vi "créer code EMBALLAGE_ZEBRA_3844Z.vi"(0 "DIVISION":enum16{"FLATPROP", "MEDIC"}(ring)=enum."MEDIC", 1 "N° carton":u8=1, 2 "DATA cmde":T1={"n°article FAS"="12-216C-04521 EQIFIL 417mA 14.4ohm", "n° cmde FAS"="03838/08-01.07.01", "quantité cmde"="100", "ID LIG cmde"="966584", "n° cmde client"="CF-08-0253/2", "nom client"="EMS Electro Medical System", "n° article client"="EL-360", "indice revision client"="03", "société de facturation"="FAS Medic", "langue a utiliser"="FR"}, 3 "Nb total cartons":i32, 9 "Tableau n° valves":string[](array[string])=["112105740008010001", "112105740008010002", "112105740008010003", "112105740008010004", "112105740008010005", "112105740008010006", "112105740008010007", "112105740008010008", "112105740008010009", "112105740008010010", "112105740008010011", "112105740008010012", "112105740008010013", "112105740008010014", "112105740008010015", "112105740008010016", "112105740008010017", "112105740008010018", "112105740008010019", "112105740008010020", "112105740008010021", "112105740008010022", "112105740008010023", "112105740008010024", "112105740008010025", "112105740008010026", "112105740008010027", "112105740008010028", "112105740008010029", "112105740008010030", "112105740008010031", "112105740008010032", "112105740008010033", "112105740008010034", "112105740008010035", "112105740008010036", "112105740008010037", "112105740008010038", "112105740008010039", "112105740008010040", "112105740008010041", "112105740008010042", "112105740008010043", "112105740008010044", "112105740008010045", "112105740008010046", "112105740008010047", "112105740008010048", "112105740008010049", "112105740008010050"], 11 "error in (no error)":errorcluster caption="entrée d'erreur (pas d'erreur)", 12 "Tableau \nlots OUT":string[][](array[string])) -> (6 "chaine  à écrire":string="^XA\n^KL3\n^SC9600,8,N,1,,N\n^PRA\n^LL1428\n^ML888\n^MMC\n^LH100,90\r\r^AFB,1,1^FT0,940^FDDestinataire : EMS Electro Medical System^FS\r^AFB,1,1^FT40,940^FDN§ commande : CF-08-0253/2^FS\r^AFB,1,1^FT80,940^FDQuantit‚ : 50/100^FS\r^AFB,1,1^FT120,940^FDVotre r‚f. : EL-360^FS\r^AFB,1,1^FT200,940^FDN§ valves :^FS\r^AFB,1,1^FT235,905^FD(P/N)^FS\r\r^FT588,30\n^BY2,2.0\n^BCI,80,N,N,N\n^FDEL-360 03 08010801 50^FS\r^A0I,30,30^FT441,0^FDEL-360 03 08010801 50^FS\r\r^A0B,24,24^FT200,750^FD  08010001,  08010002,  08010003,  08010004,  08010005^FS\r^A0B,24,24^FT225,750^FD  08010006,  08010007,  08010008,  08010009,  08010010^FS\r^A0B,24,24^FT250,750^FD  08010011,  08010012,  08010013,  08010014,  08010015^FS\r^A0B,24,24^FT275,750^FD  08010016,  08010017,  08010018,  08010019,  08010020^FS\r^A0B,24,24^FT300,750^FD  08010021,  08010022,  08010023,  08010024,  08010025^FS\r^A0B,24,24^FT325,750^FD  08010026,  08010027,  08010028,  08010029,  08010030^FS\r^A0B,24,24^FT350,750^FD  08010031,  08010032,  08010033,  08010034,  08010035^FS\r^A0B,24,24^FT375,750^FD  08010036,  08010037,  08010038,  08010039,  08010040^FS\r^A0B,24,24^FT400,750^FD  08010041,  08010042,  08010043,  08010044,  08010045^FS\r^A0B,24,24^FT425,750^FD  08010046,  08010047,  08010048,  08010049,  08010050^FS\r\r^FT465,940\n^GB0,800,3^FS\n\n^FT650,940\n^BXB,6,0\n^FD12-216C-04521 EQIFIL 417mA 14.4ohm;03838/08-01.07.01;1/2^FS\r^AFB,1,1^FT525,760^FDN§ article FAS :^FS\r^A0B,30,30^FT560,760^FD12-216C-04521 EQIFIL 417mA 14.4ohm^FS\r^AFB,1,1^FT595,760^FDN§ commande FAS :^FS\r^A0B,30,30^FT630,760^FD03838/08-01.07.01^FS\r^AFB,1,1^FT665,760^FDCarton : ^FS\r^A0B,30,30^FT665,616^FD1/2^FS\r\r^PQ1\n^XZ\r", 8 "Dec.Droite":string="^LH70,20", 10 "n°article FAS":string, 15 "error out":errorcluster caption="sortie d'erreur")   [LabVIEW 2020]
doc: "Crée le code à envoyer à l'imprimante\nFormat : Carton 1/1 dans le code bar 2D"
uses:
  Modules/FS/60_FS_Controles/60_FS_SetGet.ctl
panel:
  out "S122.0009":bool
  out "RETOUR ?":bool
  out "ligne10":string=" 08010046,  08010047,  08010048,  08010049,  08010050"
  out "ligne9":string=" 08010041,  08010042,  08010043,  08010044,  08010045"
  out "ligne8":string=" 08010036,  08010037,  08010038,  08010039,  08010040"
  out "ligne7":string=" 08010031,  08010032,  08010033,  08010034,  08010035"
  out "ligne6":string=" 08010026,  08010027,  08010028,  08010029,  08010030"
  out "ligne5":string=" 08010021,  08010022,  08010023,  08010024,  08010025"
  out "ligne4":string=" 08010016,  08010017,  08010018,  08010019,  08010020"
  out "ligne3":string=" 08010011,  08010012,  08010013,  08010014,  08010015"
  out "ligne2":string=" 08010006,  08010007,  08010008,  08010009,  08010010"
  out "ligne1":string=" 08010001,  08010002,  08010003,  08010004,  08010005"
  out "Ref client":string="EL-360"
  out "Quantité":string="50/100"
  out "carton":string="1/2"
  out "N° cmde client":string="CF-08-0253/2"
  out "Nom client":string="EMS Electro Medical System"
  out "nom valve FAS":string="12-216C-04521 EQIFIL 417mA 14.4ohm"
  out "n° commande FAS":string="03838/08-01.07.01"
  out "nom sous code bar client":string="EL-360 03 08010801 50"
  # "^XA\n^KL3\n^SC9600,8,N,1,,N\n^PRA\n^LL976\n^ML592\n^LH25,25\n\n^ADB,1,1^FT25,704^FDDestinataire :  EMS Electro Medical System^FS\n^ADB,1,1^FT50,704^FDN§ commande : CF-08-0253/2^FS\n^ADB,1,1^FT75,704^FDCarton : 1/2^FS\n^ADB,1,1^FT100,704^FDQuantit‚ : 50/100^FS\n^ADB,1,1^FT125,704^FDVotre r‚f. : EL-360^FS\n\n^ADB,1,1^FT180,704^FDN§ valves :^FS\n^ADB,1,1^FT205,678^FD(P/N)^FS\n^A0B,18,18^FT180,568^FD 08120001,  08120002,  08120003,  08120004,  08120005^FS\n^A0B,18,18^FT198,568^FD 08120006,  08120007,  08120008,  08120009,  08120010^FS\n^A0B,18,18^FT216,568^FD 08120011,  08120012,  08120013,  08120014,  08120015^FS\n^A0B,18,18^FT234,568^FD 08120016,  08120017,  08120018,  08120019,  08120020^FS\n^A0B,18,18^FT252,568^FD 08120021,  08120022,  08120023,  08120024,  08120025^FS\n^A0B,18,18^FT270,568^FD 08120026,  08120027,  08120028,  08120029,  08120030^FS\n^A0B,18,18^FT288,568^FD 08120031,  08120032,  08120033,  08120034,  08120035^FS\n^A0B,18,18^FT306,568^FD 08120036,  08120037,  08120038,  08120039,  08120040^FS\n^A0B,18,18^FT324,568^FD 08120041,  08120042,  08120043,  08120044,  08120045^FS\n^A0B,18,18^FT342,568^FD 08120046,  08120047,  08120048,  08120049,  08120050^FS\n\n^FT370,708\n^GB0,565,3^FS\n\n^FT501,708\n^BXB,4,0\n^FD12-216C-04521 EQIFIL 417mA 14.4ohm     03838/08-07.01.01^FS\n\n^ADB,1,1^FT413,568^FDN§ article FAS :^FS\n^AQB,1,1^FT443,568^FD12-216C-04521 EQIFIL 417mA 14.4ohm^FS\n^ADB,1,1^FT470,568^FDN§ commande FAS :^FS\n^AQB,1,1^FT500,568^FD03838/08-07.01.01^FS\n\n^FT352,40\n^BY1,2.0\n^BCI,56,N,N,N\n^FDEL-360 03 08120812 50^FS\n^AQI,1,1^FT352,10^FDEL-360 03 08120812 50^FS\n\n^PQ1\n^XZ"
  # "Destinataire:"
  # "N°commande :"
  # "Quantité:"
  # "Votre ref.:"
  # "N° valves :\n(P/N)"
  # "N°article FAS:"
  # "N°commande FAS:"
  # "Carton :"
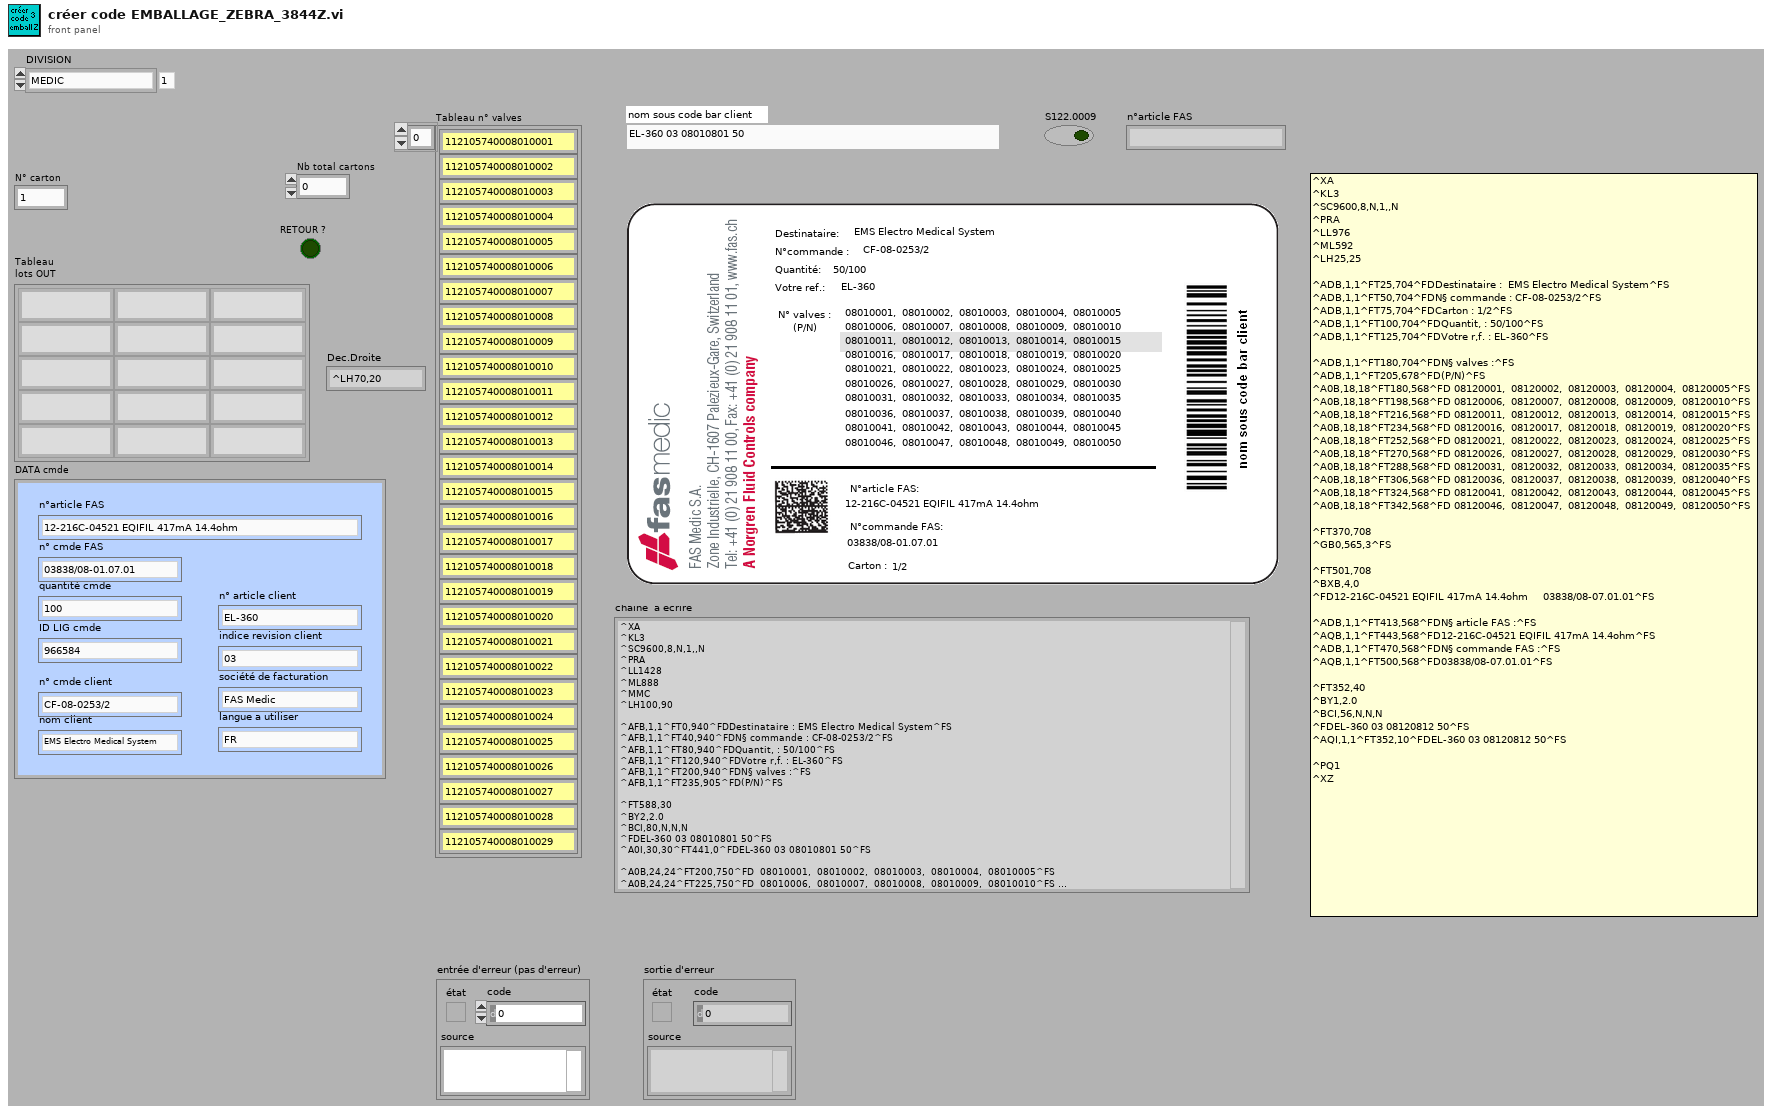
[diagram p1: front panel]
types:
  T1 = typedef "DATA commande.ctl" = cluster{"n°article FAS":string, "n° cmde FAS":string, "quantité cmde":string, "ID LIG cmde":string, "n° cmde client":string, "nom client":string, "n° article client":string, "indice revision client":string, "société de facturation":string, "langue a utiliser":string}
  T2 = typedef "60_FS_SetGet.ctl" = enum16{"set", "get"}
  T3 = typedef "Emballage_BDD_param_Produit.ctl" = cluster{"No_Valve_FAS":string, "suffixe":string, "designation":string, "indice_produit":string, "code_barre_fixe":string, "affiche_code_barre_client":string, "affiche_no_client":string, "Nb_vlve_par_carton":u16, "melange_des_lots_possible":string, "id_article":string, "Indice_Rev":string, "Famille":string, "date":string, "code_barre_fixe_Fin":string, "Longeur_No_Serie":string}
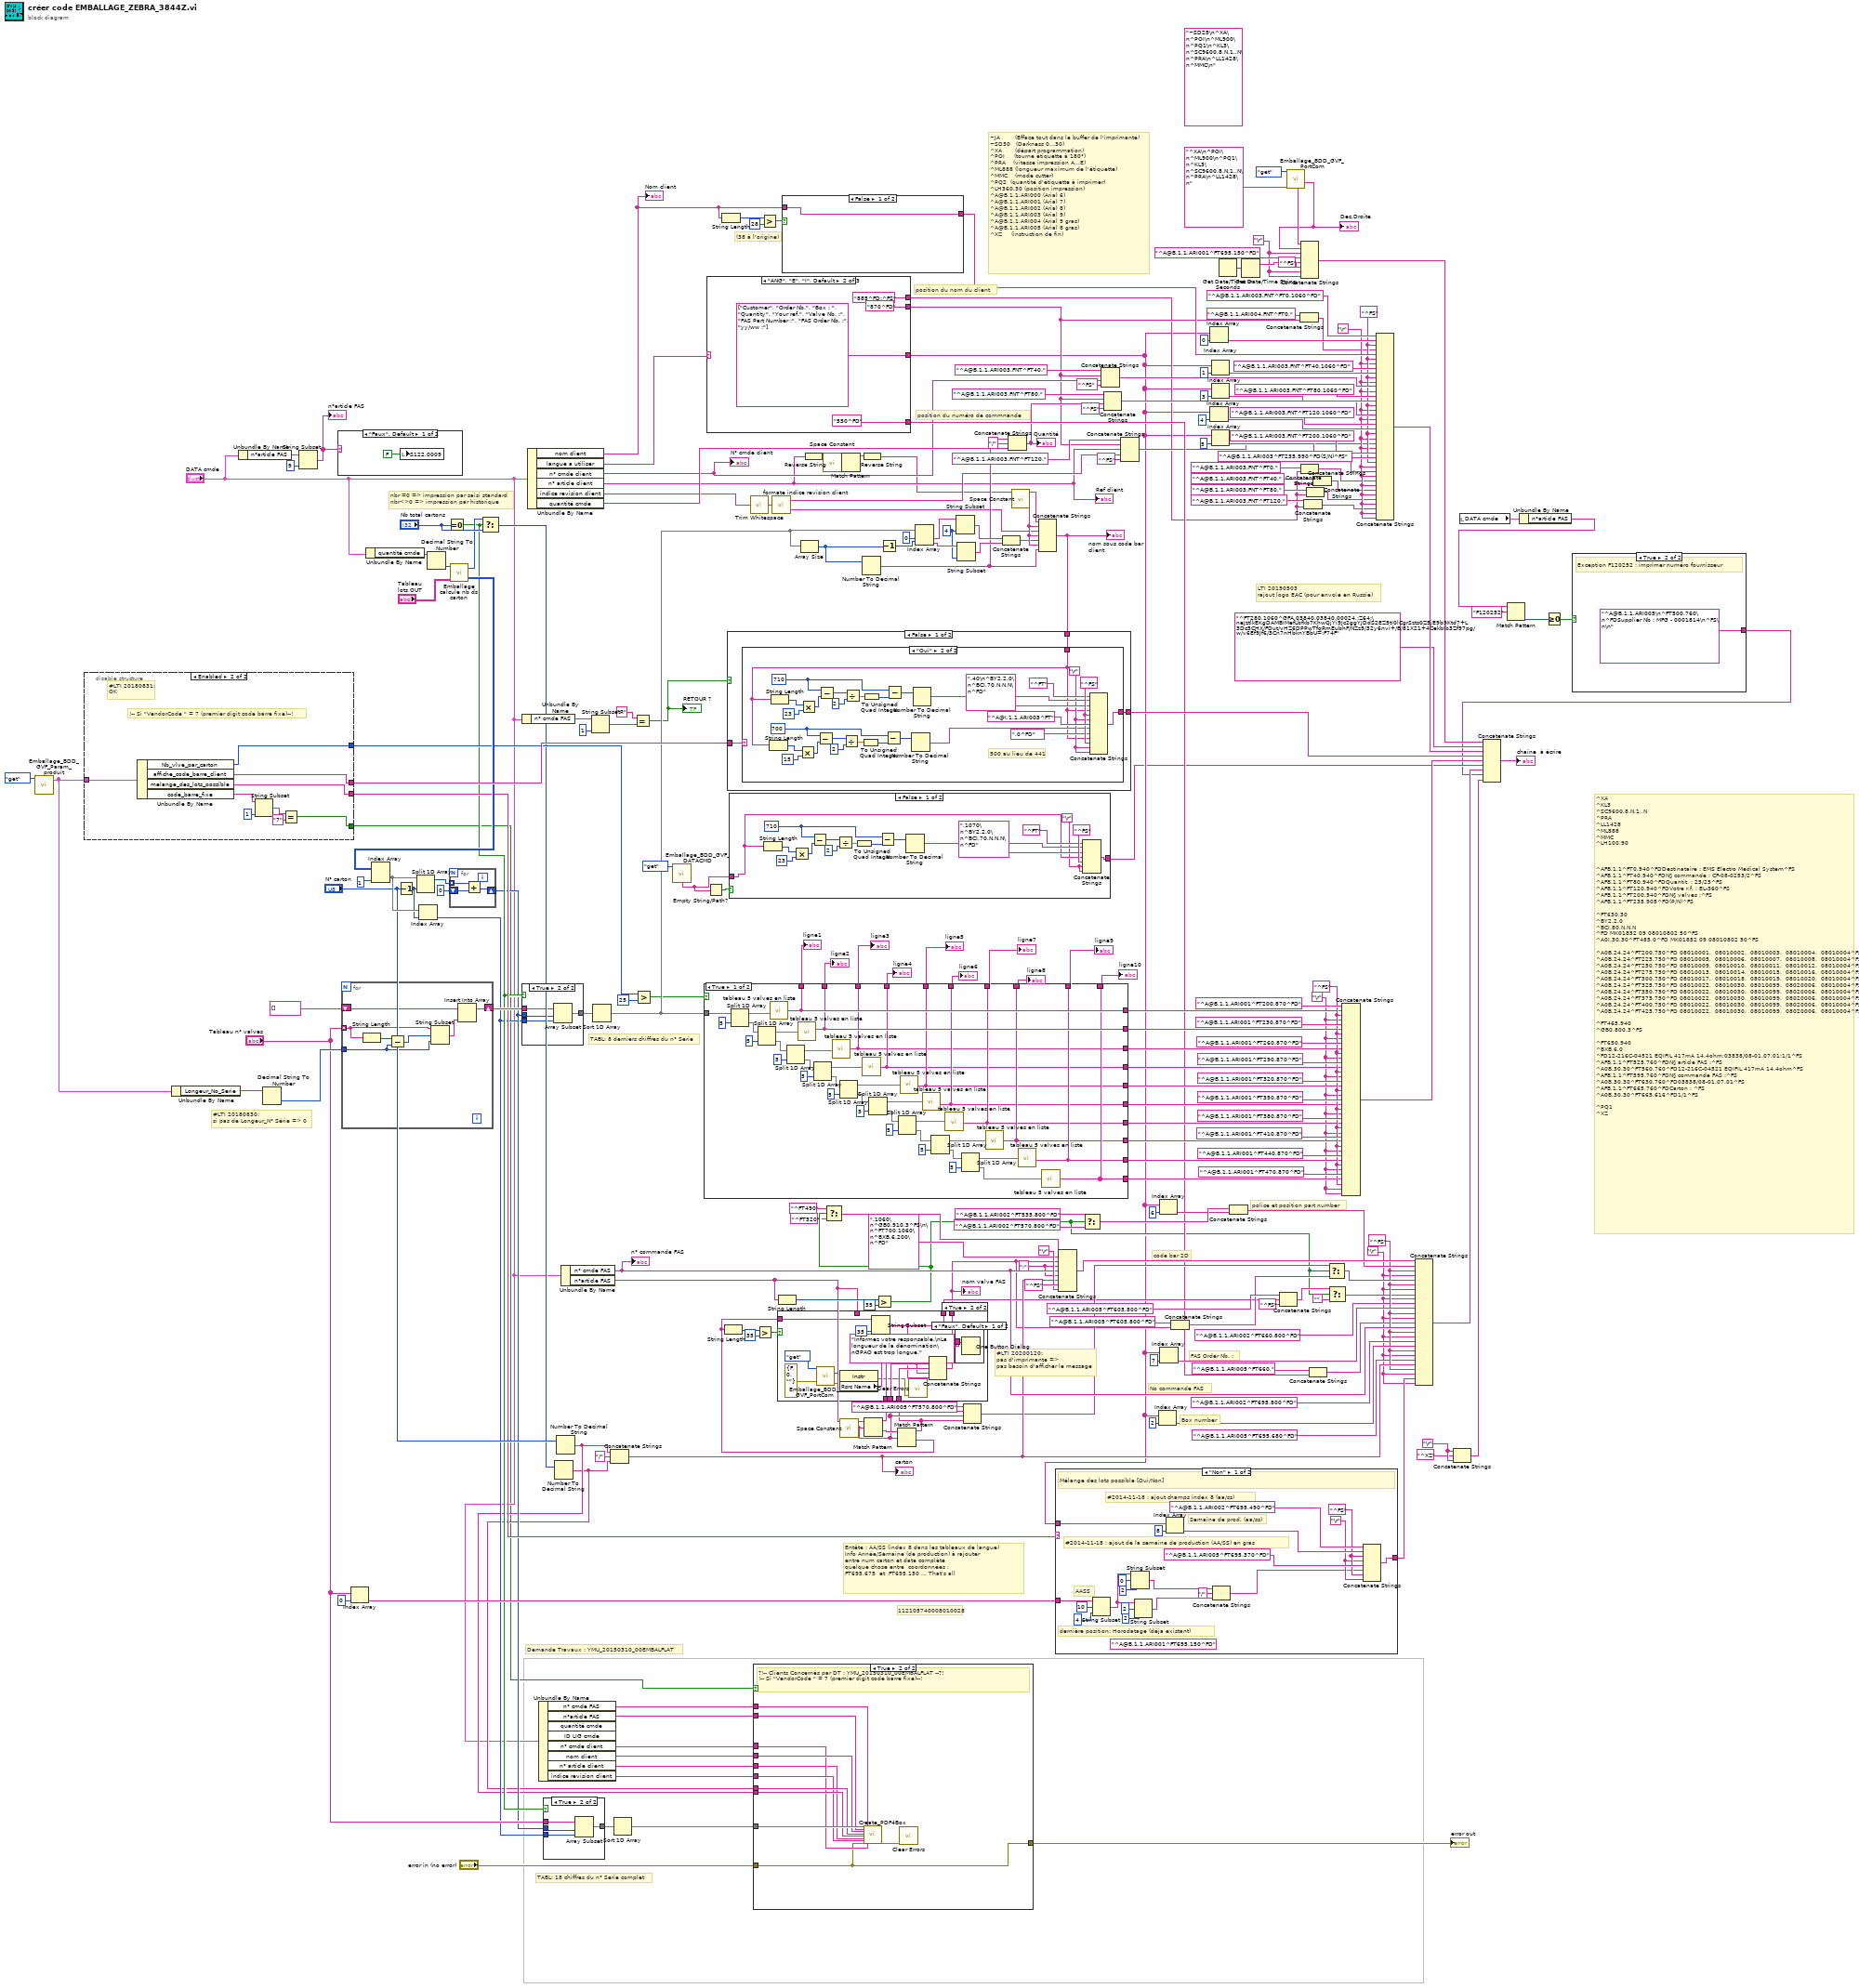
[diagram p0: block diagram]
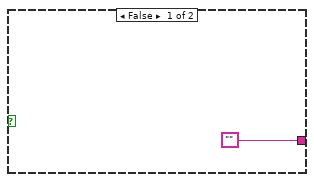
[diagram p2: hidden frame]
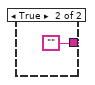
[diagram p3: hidden frame]
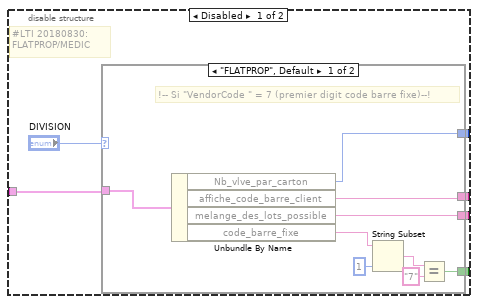
[diagram p4: hidden frame]
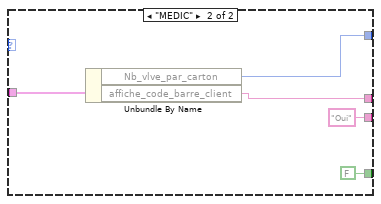
[diagram p5: hidden frame]
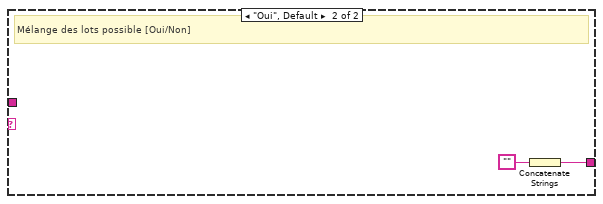
[diagram p8: hidden frame]
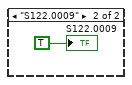
[diagram p9: hidden frame]
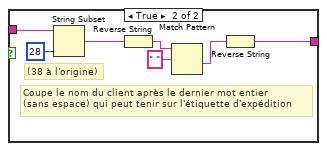
[diagram p11: hidden frame]
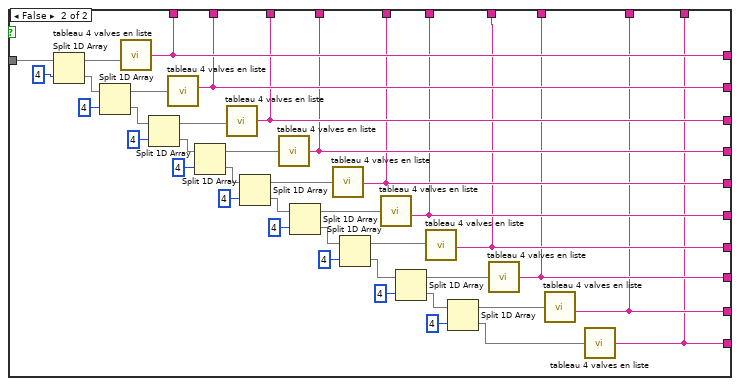
[diagram p14: hidden frame]
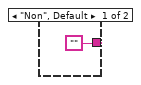
[diagram p15: hidden frame]
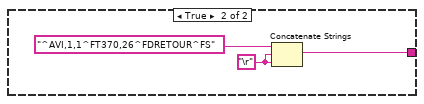
[diagram p16: hidden frame]
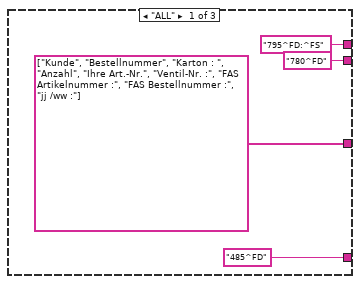
[diagram p17: hidden frame]
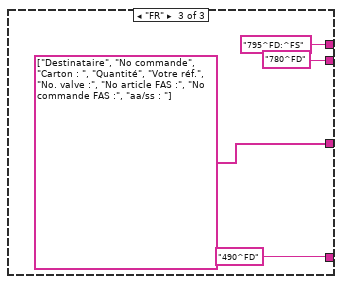
[diagram p18: hidden frame]
diagram:
  (unwired) "~SD25\n^XA\n^POI\n^ML900\n^PQ1\n^KL3\n^SC9600,8,N,1,,N\n^PRA\n^LL1428\n^MMC\n"
  w119 = "\r"
  w41 = "\r"
  w123 = "^FS"
  w144 = ";"
  w203 = "^FS"
  w164 = "\r"
  w94 = "^FS"
  w93 = "\r"
  w48 = "\r"
  w234 = 4 ("longueur (reste)")
  # "#LTI 20200120:\npas d'imprimante =>\npas besoin d'afficher le message"
  # "LTI 20190503\nrajout logo EAC (pour envoie en Russie)"
  # "#LTI 20180830:\nsi pas de Longeur_N° Série => 0"
  # "Demande Travaux : YMU_20150310_00EMBALFLAT"
  # "TABL: 18 chiffres du n° Serie complet"
  # "TABL: 8 derniers chiffres du n° Serie"
  # "112105740008010028"
  # "Entête : AA/SS (index 8 dans les tableaux de langue)\nInfo Année/Semaine (de production) à rajouter \nentre num carton et date complète\nquelque chose entre  coordonnées :      \nFT695,675  et  FT695,150 ... That's all"
  # "(38 à l'origine)"
  # "nbr =0 => impression par saisi standard\nnbr<>0 => impression par historique"
  # "position du numéro de commnande"
  # "position du nom du client"
  # "Box number"
  # "No commande FAS"
  # "FAS Order Nb. :"
  # "police et position part number"
  # "code bar 2D"
  # "~JA        (Efface tout dans le buffer de l'imprimante)\n~SD30   (Darkness 0...30)\n^XA       (départ programmation)\n^POI     (tourne étiquette à 180°)\n^PRA    (vitesse impression A...E)\n^ML888 (longueur maximum de l'étiquette)\n^MMC    (mode cutter)\n^PQ2  (quantité d'étiquette à imprimer)\n^LH360,30 (position impression)\n^A@B,1,1,ARI000 (Arial 6)\n^A@B,1,1,ARI001 (Arial 7)\n^A@B,1,1,ARI002 (Arial 8)\n^A@B,1,1,ARI003 (Arial 9)\n^A@B,1,1,ARI004 (Arial 9 gras)\n^A@B,1,1,ARI005 (Arial 8 gras)\n^XZ     (instruction de fin)"
  # "^XA\n^KL3\n^SC9600,8,N,1,,N\n^PRA\n^LL1428\n^ML888\n^MMC\n^LH100,90\n\n\n\n^AFB,1,1^FT0,940^FDDestinataire : EMS Electro Medical System^FS\n^AFB,1,1^FT40,940^FDN§ commande : CF-08-0253/2^FS\n^AFB,1,1^FT80,940^FDQuantit‚ : 25/25^FS\n^AFB,1,1^FT120,940^FDVotre r‚f. : EL-360^FS\n^AFB,1,1^FT200,940^FDN§ valves :^FS\n^AFB,1,1^FT235,905^FD(P/N)^FS\n\n^FT630,30\n^BY2,2.0\n^BCI,80,N,N,N\n^FD MK01852 09 08010802 50^FS\n^A0I,30,30^FT485,0^FD MK01852 09 08010802 50^FS\n\n^A0B,24,24^FT200,750^FD 08010001,  08010002,  08010003,  08010004,  08010004^FS\n^A0B,24,24^FT225,750^FD 08010005,  08010006,  08010007,  08010008,  08010004^FS\n^A0B,24,24^FT250,750^FD 08010009,  08010010,  08010011,  08010012,  08010004^FS\n^A0B,24,24^FT275,750^FD 08010013,  08010014,  08010015,  08010016,  08010004^FS\n^A0B,24,24^FT300,750^FD 08010017,  08010018,  08010019,  08010020,  08010004^FS\n^A0B,24,24^FT325,750^FD 08010022,  08010030,  08010099,  08020006,  08010004^FS\n^A0B,24,24^FT350,750^FD 08010022,  08010030,  08010099,  08020006,  08010004^FS\n^A0B,24,24^FT375,750^FD 08010022,  08010030,  08010099,  08020006,  08010004^FS\n^A0B,24,24^FT400,750^FD 08010022,  08010030,  08010099,  08020006,  08010004^FS\n^A0B,24,24^FT425,750^FD 08010022,  08010030,  08010099,  08020006,  08010004^FS\n\n^FT465,940\n^GB0,800,3^FS\n\n^FT650,940\n^BXB,6,0\n^FD12-216C-04521 EQIFIL 417mA 14.4ohm;03838/08-01.07.01;1/1^FS\n^AFB,1,1^FT525,760^FDN§ article FAS :^FS\n^A0B,30,30^FT560,760^FD12-216C-04521 EQIFIL 417mA 14.4ohm^FS\n^AFB,1,1^FT595,760^FDN§ commande FAS :^FS\n^A0B,30,30^FT630,760^FD03838/08-01.07.01^FS\n^AFB,1,1^FT665,760^FDCarton : ^FS\n^A0B,30,30^FT665,616^FD1/1^FS\n\n^PQ1\n^XZ"
  n1 = call "Emballage_BDD_GVF_Param_produit.vi"("Énum"=enum16{"set", "get"}."get") -> ("CLS_param_produit"=w17:T3)  [unwired: 7 in, 3 out]
  n2 = disable-structure shown="Enabled" {
    disable-tunnel: [w245 w261] -> w189
    disable-tunnel: [w244 w260] -> w150
    disable-tunnel: [w243 w262] -> w44
    disable-tunnel: [w242 w264] -> w21
    disable-tunnel: w17 -> [w241 w263]
    frame Disabled {
      # "#LTI 20180830:\nFLATPROP/MEDIC"
      n3 = case shown="\"FLATPROP\", Default" "DIVISION" {
        tunnel: [w253 w256] -> w245
        tunnel: [w254 w255] -> w244
        tunnel: w241 -> [w252 w257]
        tunnel: [w251 "Oui" ("Mélange des lots posiible [Oui/Non]")] -> w243
        tunnel: [w246 FALSE] -> w242
        frame "FLATPROP", Default {
          # "!-- Si \"VendorCode \" = 7 (premier digit code barre fixe)--!"
          n4 = Unbundle By Name(w252) -> ("Nb_vlve_par_carton"=w254:u16, "affiche_code_barre_client"=w253:string, "melange_des_lots_possible"=w251:string, "code_barre_fixe"=w250:string)
          n5 = String Subset(string=w250, length (rest)=1 ("longueur (reste)")) -> (substring=w248:string)  [unwired: 1 in]
          n6 = Equal?(x=w248, y="7") -> (x = y?=w246:bool)
        }
        frame "MEDIC" {
          n7 = Unbundle By Name(w257) -> ("Nb_vlve_par_carton"=w255:u16, "affiche_code_barre_client"=w256:string)
        }
      }
    }
    frame Enabled {
      # "#LTI 20180831:\nOK"
      # "!-- Si \"VendorCode \" = 7 (premier digit code barre fixe)--!"
      n8 = Unbundle By Name(w263) -> ("Nb_vlve_par_carton"=w260:u16, "affiche_code_barre_client"=w261:string, "melange_des_lots_possible"=w262:string, "code_barre_fixe"=w268:string)
      n9 = String Subset(string=w268, length (rest)=1 ("longueur (reste)")) -> (substring=w266:string)  [unwired: 1 in]
      n10 = Equal?(x=w266, y="7") -> (x = y?=w264:bool)
    }
  }
  n11 = Unbundle By Name(w17) -> ("Longeur_No_Serie"=w16:string)
  n12 = Unbundle By Name("DATA cmde") -> ("n°article FAS"=w47:string)
  n13 = Decimal String To Number(string=w16) -> (number=w50:i32)  [unwired: 2 in, 1 out]
  n14 = String Subset(string=w47, length (rest)=9 ("longueur (reste)")) -> (substring=w45:string)  [unwired: 1 in]
  "n°article FAS" <- w45
  n15 = case shown="\"Faux\", Default" w45 {
    frame "Faux", Default {
      n16 = local write "S122.0009"(FALSE ("S122.0009")) -> ()
    }
    frame "S122.0009" {
      "S122.0009" <- TRUE ("S122.0009")
    }
  }
  n17 = for {
    tunnel: "Tableau n° valves" -> [w274] mode=indexing
    shift-right: [w276] -> w185
    shift-left: string[] [] -> [w275]
    tunnel: w50 -> [w271]
    n18 = String Length(string=w274) -> (length=w273:i32)
    n19 = Subtract(x=w273, y=w271) -> (x-y=w272:i32)
    n20 = String Subset(string=w274, offset (0)=w272, length (rest)=w271) -> (substring=w277:string)
    n21 = Insert Into Array(array=w275, new element=w277) -> (w276:string[])  [unwired: 1 in]
  }
  n22 = Index Array(array="Tableau n° valves", index=0 ("indice")) -> (element=w39:string)
  n23 = Unbundle By Name("DATA cmde") -> ("quantité cmde"=w19:string)
  n24 = Decrement(x="N° carton") -> (x-1=w180:u8)
  n25 = Decimal String To Number(string=w19) -> (number=w18:i32)  [unwired: 2 in, 1 out]
  n26 = Equal To 0?(x="Nb total cartons") -> (x = 0?=w36:bool)
  n27 = call "Emballage calcule nb ds carton.vi"("Tableau \nlots OUT"="Tableau \nlots OUT", "Quantité de la cmde"=w18) -> ("Tab n° carton - nb ds carton"=w177:i32[][], "Nb total cartons"=w59:i32)  [unwired: 1 in]
  n28 = Index Array(array=w177, index (col)=1 ("indice désactivé (col)")) -> (element=w181:i32[])  [unwired: 1 in]
  n29 = Split 1D Array(array=w181, index=w180) -> (first subarray=w182:i32[])  [unwired: 1 out]
  n30 = Index Array(array=w181, index=w180) -> (element=w34:i32)
  n31 = for {
    tunnel: w182 -> [w280] mode=indexing
    shift-right: [w278] -> w35
    shift-left: 0 -> [w279]
    n32 = Add(x=w280, y=w279) -> (x+y=w278:i32)
  }
  n33 = Select(t=w59, s=w36, f="Nb total cartons") -> (s? t:f=w58:i32)
  n34 = Unbundle By Name("DATA cmde") -> ("n° cmde FAS"=w149:string)
  n35 = case shown="True" w36 {
    tunnel: w185 -> [w281 w285]
    tunnel: [w281 w284] -> w184
    tunnel: w35 -> [_ w283]
    tunnel: w34 -> [_ w282]
    frame False {
    }
    frame True {
      n36 = Array Subset(array=w285, index=w283, length=w282) -> (w284:string[])
    }
  }
  n37 = Unbundle By Name("DATA cmde") -> ("nom client"=w112:string, "langue a utiliser"=w191:string, "n° cmde client"=w100:string, "n° article client"=w55:string, "indice revision client"=w56:string, "quantité cmde"=w190:string)
  "Nom client" <- w112
  "N° cmde client" <- w100
  "Ref client" <- w55
  n38 = Unbundle By Name("DATA cmde") -> ("n° cmde FAS"=w29:string, "n°article FAS"=w28:string, "n° cmde client"=w26:string, "nom client"=w22:string, "n° article client"=w25:string, "indice revision client"=w27:string)  [unwired: 2 out]
  n39 = case shown="True" w36 {
    tunnel: "Tableau n° valves" -> [w286 w290]
    tunnel: [w286 w289] -> w38
    tunnel: w35 -> [_ w288]
    tunnel: w34 -> [_ w287]
    frame False {
    }
    frame True {
      n40 = Array Subset(array=w290, index=w288, length=w287) -> (w289:string[])
    }
  }
  n41 = Number To Decimal String(number=w58) -> (decimal integer string=w31:string)  [unwired: 1 in]
  n42 = Number To Decimal String(number="N° carton") -> (decimal integer string=w32:string)  [unwired: 1 in]
  n43 = Unbundle By Name("DATA cmde") -> ("n° cmde FAS"=w175:string, "n°article FAS"=w107:string)
  "n° commande FAS" <- w175
  n44 = String Subset(string=w149, length (rest)=1 ("longueur (reste)")) -> (substring=w146:string)  [unwired: 1 in]
  n45 = Sort 1D Array(array=w184) -> (sorted array=w178:string[])
  n46 = Concatenate Strings(w32, "/", w31) -> (w141:string)
  "carton" <- w141
  n47 = Sort 1D Array(array=w38) -> (sorted array=w33:string[])
  n48 = Equal?(x="R", y=w146) -> (x = y?=w147:bool)
  "RETOUR ?" <- w147
  n49 = Greater?(x=w150, y=u16 25) -> (0:w152:bool)
  n50 = call "Emballage_BDD_GVF_DATACMD.vi"("SetGet"=60_FS_SetGet."get") -> ("NO_ARTICLE_JDE"=w10:string)  [unwired: 7 in, 7 out]
  n51 = case shown="True" w152 {
    tunnel: w178 -> [w301 w339]
    tunnel: [w300 w338] -> w174
    tunnel: [w299 w337] -> w173
    tunnel: [w291 w336] -> w172
    tunnel: [w298 w329] -> w171
    tunnel: [w297 w330] -> w170
    tunnel: [w296 w331] -> w169
    tunnel: [w295 w332] -> w168
    tunnel: [w294 w333] -> w167
    tunnel: [w293 w334] -> w166
    tunnel: [w292 w335] -> w165
    tunnel: [w300 w338] -> w162
    tunnel: [w299 w337] -> w161
    tunnel: [w298 w329] -> w160
    tunnel: [w297 w330] -> w159
    tunnel: [w296 w331] -> w158
    tunnel: [w295 w332] -> w157
    tunnel: [w294 w333] -> w156
    tunnel: [w293 w334] -> w155
    tunnel: [w292 w335] -> w154
    tunnel: [w291 w336] -> w153
    frame True {
      n52 = Split 1D Array(array=w301, index=5 ("indice")) -> (first subarray=w319:string[], second subarray=w326:string[])
      n53 = Split 1D Array(array=w326, index=5 ("indice")) -> (first subarray=w318:string[], second subarray=w324:string[])
      n54 = call "tableau 5 valves en liste.vi"("Tableau de 5 valves"=w319) -> ("Chaîne de 5 valves"=w300:string)
      n55 = Split 1D Array(array=w324, index=5 ("indice")) -> (first subarray=w317:string[], second subarray=w322:string[])
      n56 = call "tableau 5 valves en liste.vi"("Tableau de 5 valves"=w318) -> ("Chaîne de 5 valves"=w299:string)
      n57 = Split 1D Array(array=w322, index=5 ("indice")) -> (first subarray=w316:string[], second subarray=w320:string[])
      n58 = call "tableau 5 valves en liste.vi"("Tableau de 5 valves"=w317) -> ("Chaîne de 5 valves"=w291:string)
      n59 = Split 1D Array(array=w320, index=5 ("indice")) -> (first subarray=w315:string[], second subarray=w313:string[])
      n60 = call "tableau 5 valves en liste.vi"("Tableau de 5 valves"=w316) -> ("Chaîne de 5 valves"=w292:string)
      n61 = Split 1D Array(array=w313, index=5 ("indice")) -> (first subarray=w312:string[], second subarray=w310:string[])
      n62 = Split 1D Array(array=w310, index=5 ("indice")) -> (first subarray=w309:string[], second subarray=w307:string[])
      n63 = call "tableau 5 valves en liste.vi"("Tableau de 5 valves"=w315) -> ("Chaîne de 5 valves"=w293:string)
      n64 = call "tableau 5 valves en liste.vi"("Tableau de 5 valves"=w312) -> ("Chaîne de 5 valves"=w294:string)
      n65 = Split 1D Array(array=w307, index=5 ("indice")) -> (first subarray=w306:string[], second subarray=w304:string[])
      n66 = call "tableau 5 valves en liste.vi"("Tableau de 5 valves"=w309) -> ("Chaîne de 5 valves"=w295:string)
      n67 = Split 1D Array(array=w304, index=5 ("indice")) -> (first subarray=w303:string[], second subarray=w302:string[])
      n68 = call "tableau 5 valves en liste.vi"("Tableau de 5 valves"=w306) -> ("Chaîne de 5 valves"=w296:string)
      n69 = call "tableau 5 valves en liste.vi"("Tableau de 5 valves"=w303) -> ("Chaîne de 5 valves"=w297:string)
      n70 = call "tableau 5 valves en liste.vi"("Tableau de 5 valves"=w302) -> ("Chaîne de 5 valves"=w298:string)
    }
    frame False {
      n71 = Split 1D Array(array=w339, index=4 ("indice")) -> (first subarray=w357:string[], second subarray=w364:string[])
      n72 = Split 1D Array(array=w364, index=4 ("indice")) -> (first subarray=w356:string[], second subarray=w362:string[])
      n73 = call "tableau 4 valves en liste.vi"("Tableau de 4 valves"=w357) -> ("Chaîne de 5 valves"=w338:string)
      n74 = Split 1D Array(array=w362, index=4 ("indice")) -> (first subarray=w355:string[], second subarray=w360:string[])
      n75 = call "tableau 4 valves en liste.vi"("Tableau de 4 valves"=w356) -> ("Chaîne de 5 valves"=w337:string)
      n76 = Split 1D Array(array=w360, index=4 ("indice")) -> (first subarray=w354:string[], second subarray=w358:string[])
      n77 = call "tableau 4 valves en liste.vi"("Tableau de 4 valves"=w355) -> ("Chaîne de 5 valves"=w336:string)
      n78 = Split 1D Array(array=w358, index=4 ("indice")) -> (first subarray=w353:string[], second subarray=w351:string[])
      n79 = call "tableau 4 valves en liste.vi"("Tableau de 4 valves"=w354) -> ("Chaîne de 5 valves"=w335:string)
      n80 = Split 1D Array(array=w351, index=4 ("indice")) -> (first subarray=w350:string[], second subarray=w348:string[])
      n81 = call "tableau 4 valves en liste.vi"("Tableau de 4 valves"=w353) -> ("Chaîne de 5 valves"=w334:string)
      n82 = Split 1D Array(array=w348, index=4 ("indice")) -> (first subarray=w347:string[], second subarray=w345:string[])
      n83 = call "tableau 4 valves en liste.vi"("Tableau de 4 valves"=w350) -> ("Chaîne de 5 valves"=w333:string)
      n84 = Split 1D Array(array=w345, index=4 ("indice")) -> (first subarray=w344:string[], second subarray=w342:string[])
      n85 = call "tableau 4 valves en liste.vi"("Tableau de 4 valves"=w347) -> ("Chaîne de 5 valves"=w332:string)
      n86 = Split 1D Array(array=w342, index=4 ("indice")) -> (first subarray=w341:string[], second subarray=w340:string[])
      n87 = call "tableau 4 valves en liste.vi"("Tableau de 4 valves"=w344) -> ("Chaîne de 5 valves"=w331:string)
      n88 = call "tableau 4 valves en liste.vi"("Tableau de 4 valves"=w341) -> ("Chaîne de 5 valves"=w330:string)
      n89 = call "tableau 4 valves en liste.vi"("Tableau de 4 valves"=w340) -> ("Chaîne de 5 valves"=w329:string)
    }
  }
  "ligne1" <- w162
  "ligne2" <- w161
  "ligne3" <- w153
  "ligne4" <- w154
  "ligne5" <- w155
  "ligne6" <- w156
  "ligne7" <- w157
  "ligne8" <- w158
  "ligne9" <- w159
  "ligne10" <- w160
  n90 = case shown="\"ANG\", \"E\", \"I\", Default" w191 {
    tunnel: [string[] ["Kunde", "Bestellnummer", "Karton : ", "Anzahl", "Ihre Art.-Nr.", "Ventil-Nr. :", "FAS Artikelnummer :", "FAS Bestellnummer :", "jj /ww :"] string[] ["Customer", "Order Nb.", "Box : ", "Quantity", "Your ref.", "Valve Nb. :", "FAS Part Number :", "FAS Order Nb. :", "yy/ww :"] string[] ["Destinataire", "No commande", "Carton : ", "Quantité", "Votre réf.", "No. valve :", "No article FAS :", "No commande FAS :", "aa/ss : "]] -> w43
    tunnel: ["485^FD" "550^FD" "490^FD"] -> w101
    tunnel: ["795^FD:^FS" "885^FD:^FS" "795^FD:^FS"] -> w78
    tunnel: ["780^FD" "870^FD" "780^FD"] -> w87
    frame "ALL" {
    }
    frame "ANG", "E", "I", Default {
    }
    frame "FR" {
    }
  }
  n91 = Empty String/Path?(string/path=w10) -> (empty?=w11:bool)
  n92 = String Length(string=w112) -> (length=w114:i32)
  n93 = case shown="False" w11 {
    tunnel: [w381 ""] -> w9
    tunnel: w10 -> [w380 _]
    frame False {
      w388 = 710
      w379 = "\r"
      n94 = String Length(string=w380) -> (length=w393:i32)
      n95 = Multiply(x=w393, y=23) -> (x*y=w391:i32)
      n96 = Subtract(x=w388, y=w391) -> (x-y=w390:i32)
      n97 = Divide(x=w390, y=2) -> (x/y=w387:dbl)
      n98 = To Unsigned Quad Integer(1:w387) -> (0:w386:u64)
      n99 = Subtract(x=w388, y=w386) -> (x-y=w385:u64)
      n100 = Number To Decimal String(number=w385) -> (decimal integer string=w382:string)  [unwired: 1 in]
      n101 = Concatenate Strings("^FT", w382, ",1070\n^BY2,2.0\n^BCI,70,N,N,N\n^FD", w380, "^FS", w379, w379) -> (w381:string)
    }
    frame True {
    }
  }
  n102 = call <vilib>:"Trim Whitespace.vi"("string"=w56) -> ("trimmed string"=w57:string)  [unwired: 1 in]
  n103 = case shown="True" w21 {
    tunnel: w33 -> [_ w407]
    tunnel: w32 -> [_ w406]
    tunnel: w31 -> [_ w405]
    tunnel: w29 -> [_ w404]
    tunnel: w28 -> [_ w403]
    tunnel: w22 -> [_ w402]
    tunnel: w27 -> [_ w401]
    tunnel: w26 -> [_ w400]
    tunnel: w25 -> [_ w399]
    tunnel: [w396 w397] -> w24
    tunnel: "error in (no error)" -> [w396 w397]
    frame False {
      # "Clients non concernés"
    }
    frame True {
      # "?!-- Clients Concernés par DT : YMU_20150310_00EMBALFLAT --?!\n!-- Si \"VendorCode \" = 7 (premier digit code barre fixe)--!"
      n104 = call "Create_PDF4Box.vi"("Tableau de valves"=w407, "Produit"=w403, "Client"=w402, "Nombre Cartons"=w405, "Numero Carton"=w406, "Cust_Prod_Ref"=w399, "Cust_Indice"=w401, "error in (no error)"=w397, "Commande"=w404, "Cust_Order"=w400) -> ("error out"=w398:errorcluster)  [unwired: 17 in]
      n105 = call <vilib>:"Clear Errors.vi"("error in (no error)"=w398) -> ()  [unwired: 5 in, 2 out]
    }
  }
  "error out" <- w24
  n106 = Greater?(x=w114, y=28) -> (0:w113:bool)
  n107 = call "formate indice revision client.vi"("Indice révision client IN"=w57) -> ("Indice révision client text"=w61:string, "Indice révision client OUT"=w140:string)
  n108 = String Length(string=w107) -> (length=w117:i32)
  n109 = case shown="False" w113 {
    tunnel: w112 -> [w408 w415]
    tunnel: [w408 w409] -> w111
    frame False {
    }
    frame True {
      # "(38 à l'origine)"
      # "Coupe le nom du client après le dernier mot entier \n(sans espace) qui peut tenir sur l'étiquette d'expédition"
      n110 = String Subset(string=w415, length (rest)=28 ("longueur (reste)")) -> (substring=w410:string)  [unwired: 1 in]
      n111 = Reverse String(1:w410) -> (0:w413:string)
      n112 = Match Pattern(string=w413, regular expression=" " ("chaîne recherchée")) -> (after substring=w411:string)  [unwired: 1 in, 3 out]
      n113 = Reverse String(1:w411) -> (0:w409:string)
    }
  }
  n114 = Array Size(array=w178) -> (size(s)=w230:i32)
  n115 = Reverse String(1:w55) -> (0:w54:string)
  n116 = call <vilib>:"Space Constant.vi"() -> ("String"=w53:string)
  n117 = call <vilib>:"Space Constant.vi"() -> ("String"=w104:string)
  n118 = Match Pattern(string=w54, regular expression=w53) -> (before substring=w52:string)  [unwired: 1 in, 3 out]
  n119 = Number To Decimal String(number=w230) -> (decimal integer string=w228:string)  [unwired: 1 in]
  n120 = Reverse String(1:w52) -> (0:w51:string)
  n121 = Match Pattern(string=w107, regular expression=w104) -> (before substring=w105:string, after substring=w133:string)  [unwired: 1 in, 2 out]
  n122 = Greater?(x=w117, y=35) -> (0:w68:bool)
  n123 = Select(t="^FT490", s=w68, f="^FT520") -> (s? t:f=w69:string)
  n124 = Decrement(x=w230) -> (x-1=w231:i32)
  n125 = Match Pattern(string=w133, regular expression=w104) -> (before substring=w103:string, after substring=w109:string)  [unwired: 1 in, 2 out]
  n126 = String Length(string=w109) -> (length=w110:i32)
  n127 = Greater?(x=w110, y=35) -> (0:w116:bool)
  n128 = case shown="True" w116 {
    tunnel: w109 -> [w417 w430]
    tunnel: [w417 w425] -> w108
    tunnel: w107 -> [w416 _]
    tunnel: [w416 w424] -> w106
    tunnel: w105 -> [_ w428]
    tunnel: w104 -> [_ w426]
    tunnel: w103 -> [_ w427]
    frame False {
    }
    frame True {
      n129 = call "Emballage_BDD_GVF_PortCom.vi"("Énum"=enum16{"get", "set"}."get", "Error in"=errorcluster {"status"=FALSE, "code"=0, "source"=""}) -> ("PortCom imprimante OUT"=w422:refnum<visa-resource-name>, "Error out"=w423:errorcluster)  [unwired: 7 in, 5 out]
      n130 = property class="Instr"(reference=w422, error in=w423) -> (error out=w418:errorcluster, "Rsrc Name"=w419:string)  [unwired: 1 out]
      n131 = String Subset(string=w430, length (rest)=35 ("longueur (reste)")) -> (substring=w425:string)  [unwired: 1 in]
      n132 = call <vilib>:"Clear Errors.vi"("error in (no error)"=w418) -> ()  [unwired: 5 in, 2 out]
      n133 = Concatenate Strings(w428, w426, w427, w426, w425) -> (w424:string)
      n134 = case shown="\"Faux\", Default" w419 {
        tunnel: "Informez votre responsable.\nLa longueur de la dénomination\nGPAO est trop longue." ("message") -> [w432 _]
        frame "Faux", Default {
          n135 = One Button Dialog(message=w432) -> ()  [unwired: 1 in, 1 out]
        }
        frame "" {
        }
      }
    }
  }
  "nom valve FAS" <- w106
  n136 = Index Array(array=w178, index #1=0 ("indice"), index #2=w231) -> (element #1=w236:string, element #2=w235:string)
  n137 = String Subset(string=w236, length (rest)=w234) -> (substring=w233:string)  [unwired: 1 in]
  n138 = String Subset(string=w235, length (rest)=w234) -> (substring=w232:string)  [unwired: 1 in]
  n139 = Concatenate Strings("^A@B,1,1,ARI005^FT570,800^FD" ("chaîne"), w105, w104, w103) -> (w132:string)
  n140 = Concatenate Strings(w233, w232) -> (w237:string)
  n141 = Concatenate Strings(w228, "/" ("chaîne"), w190) -> (w97:string)
  "Quantité" <- w97
  n142 = call <vilib>:"Space Constant.vi"() -> ("String"=w238:string)
  n143 = Concatenate Strings(w51, w238, w140, w238, w237, w238, w228) -> (w76:string)
  "nom sous code bar client" <- w76
  n144 = case shown="False" w147 {
    tunnel: w76 -> [w435 _]
    tunnel: [w434 w466] -> w192
    tunnel: w189 -> [w433 _]
    frame False {
      n145 = case shown="\"Oui\"" w433 {
        tunnel: w435 -> [_ w437]
        tunnel: ["" w462] -> w434
        frame "Non", Default {
        }
        frame "Oui" {
          w444 = 700
          w456 = 710
          w463 = "^FS"
          w448 = "\r"
          # "500 au lieu de 441"
          n146 = String Length(string=w437) -> (length=w439:i32)
          n147 = String Length(string=w437) -> (length=w461:i32)
          n148 = Multiply(x=w439, y=15) -> (x*y=w441:i32)
          n149 = Multiply(x=w461, y=23) -> (x*y=w459:i32)
          n150 = Subtract(x=w444, y=w441) -> (x-y=w442:i32)
          n151 = Subtract(x=w456, y=w459) -> (x-y=w458:i32)
          n152 = Divide(x=w442, y=2) -> (x/y=w445:dbl)
          n153 = Divide(x=w458, y=2) -> (x/y=w455:dbl)
          n154 = To Unsigned Quad Integer(1:w445) -> (0:w446:u64)
          n155 = To Unsigned Quad Integer(1:w455) -> (0:w454:u64)
          n156 = Subtract(x=w444, y=w446) -> (x-y=w447:u64)
          n157 = Subtract(x=w456, y=w454) -> (x-y=w453:u64)
          n158 = Number To Decimal String(number=w447) -> (decimal integer string=w438:string)  [unwired: 1 in]
          n159 = Number To Decimal String(number=w453) -> (decimal integer string=w449:string)  [unwired: 1 in]
          n160 = Concatenate Strings("^FT", w449, ",40\n^BY2,2.0\n^BCI,70,N,N,N\n^FD", w437, w463, w448, "^A@I,1,1,ARI003^FT", w438, ",0^FD", w437, w463, w448, w448) -> (w462:string)
        }
      }
    }
    frame True {
      w467 = "\r"
      n161 = Concatenate Strings("^AVI,1,1^FT370,26^FDRETOUR^FS", w467, w467) -> (w466:string)
    }
  }
  n162 = case shown="\"Non\"" w44 {
    tunnel: [w485 w488] -> w42
    tunnel: w43 -> [w486 _]
    tunnel: w39 -> [w477 _]
    frame "Non" {
      w480 = "\r"
      w481 = "^FS"
      (unwired) "^A@B,1,1,ARI001^FT695,150^FD" ("chaîne")
      # "AASS"
      # "#2014-11-18 : ajout champs index 8 (aa/ss)"
      # "Semaine de prod. (aa/ss)"
      # "#2014-11-18 : ajout de la semaine de production (AA/SS) en gras"
      # "dernière position: Horodatage (déja existant)"
      # "Mélange des lots possible [Oui/Non]"
      n163 = String Subset(string=w477, offset (0)=10, length (rest)=4 ("longueur (reste)")) -> (substring=w472:string)
      n164 = String Subset(string=w472, offset (0)=0, length (rest)=2 ("longueur (reste)")) -> (substring=w471:string)
      n165 = String Subset(string=w472, offset (0)=2, length (rest)=2 ("longueur (reste)")) -> (substring=w470:string)
      n166 = Index Array(array=w486, index=8 ("indice")) -> (element=w483:string)
      n167 = Concatenate Strings(w471, "/" ("chaîne"), w470) -> (w468:string)
      n168 = Concatenate Strings("^A@B,1,1,ARI002^FT695,490^FD", w483, w481, w480, "^A@B,1,1,ARI005^FT695,370^FD", w468, w481, w480) -> (w485:string)
    }
    frame "Oui", Default {
      # "Mélange des lots possible [Oui/Non]"
      n169 = Concatenate Strings("") -> (w488:string)
    }
  }
  n170 = Concatenate Strings(w69, ",1060\n^GB0,910,3^FS\n\n^FT700,1060\n^BXB,6,200\n^FD", w106, w144, w175, w144, w141, "^FS", "\r") -> (w198:string)
  n171 = Select(t="^A@B,1,1,ARI002^FT535,800^FD", s=w68, f="^A@B,1,1,ARI002^FT570,800^FD") -> (s? t:f=w127:string)
  n172 = Concatenate Strings("^A@B,1,1,ARI003.FNT^FT40,", w87, w100, "^FS") -> (w99:string)
  n173 = Concatenate Strings("^A@B,1,1,ARI003.FNT^FT80,", w87, w97, "^FS") -> (w95:string)
  n174 = Concatenate Strings("^A@B,1,1,ARI003.FNT^FT120,", w87, w55, w61, "^FS") -> (w92:string)
  n175 = Index Array(array=w43, index=2 ("indice")) -> (element=w142:string)
  n176 = Index Array(array=w43, index=6 ("indice")) -> (element=w126:string)
  n177 = Index Array(array=w43, index=7 ("indice")) -> (element=w197:string)
  n178 = Concatenate Strings("^A@B,1,1,ARI005^FT605,800^FD" ("chaîne"), w106) -> (w121:string)
  n179 = Index Array(array=w43, index=0 ("indice")) -> (element=w138:string)
  n180 = Index Array(array=w43, index=4 ("indice")) -> (element=w218:string)
  n181 = Index Array(array=w43, index=1 ("indice")) -> (element=w224:string)
  n182 = Index Array(array=w43, index=3 ("indice")) -> (element=w221:string)
  n183 = Index Array(array=w43, index=5 ("indice")) -> (element=w215:string)
  n184 = Get Date/Time In Seconds() -> (seconds since 1Jan1904=w64:timestamp)
  n185 = Concatenate Strings(w127, w126) -> (w125:string)
  n186 = Get Date/Time String(seconds (now)=w64) -> (date string=w63:string)  [unwired: 2 in, 1 out]
  n187 = Concatenate Strings("^A@B,1,1,ARI005^FT605,800^FD", w108, "^FS") -> (w129:string)
  n188 = call "Emballage_BDD_GVF_PortCom.vi"("Énum"=enum16{"get", "set"}."get") -> ("DecDroit_OUT"=w13:string)  [unwired: 8 in, 6 out]
  "Dec.Droite" <- w13
  n189 = Concatenate Strings("^A@B,1,1,ARI004.FNT^FT0,", w87) -> (w86:string)
  n190 = Concatenate Strings("^XA\n^POI\n^ML900\n^PQ1\n^KL3\n^SC9600,8,N,1,,N\n^PRA\n^LL1428\n", w13, w48, "^A@B,1,1,ARI001^FT695,150^FD" ("chaîne"), w63, "^FS" ("chaîne"), w48, w48) -> (w196:string)
  n191 = Concatenate Strings("^A@B,1,1,ARI003.FNT^FT0,", w78) -> (w84:string)
  n192 = Concatenate Strings("^A@B,1,1,ARI003.FNT^FT120,", w78) -> (w77:string)
  n193 = Concatenate Strings("^A@B,1,1,ARI003.FNT^FT80,", w78) -> (w80:string)
  n194 = Concatenate Strings("^A@B,1,1,ARI005^FT660,", w101) -> (w72:string)
  n195 = Concatenate Strings("^A@B,1,1,ARI003.FNT^FT40,", w78) -> (w82:string)
  n196 = Select(t=w132, s=w68, f=w121) -> (s? t:f=w124:string)
  n197 = Select(t=w129, s=w68, f="") -> (s? t:f=w122:string)
  n198 = Concatenate Strings("^A@B,1,1,ARI001^FT200,870^FD", w174, w203, w164, "^A@B,1,1,ARI001^FT230,870^FD", w173, w203, w164, "^A@B,1,1,ARI001^FT260,870^FD", w172, w203, w164, "^A@B,1,1,ARI001^FT290,870^FD", w165, w203, w164, "^A@B,1,1,ARI001^FT320,870^FD", w166, w203, w164, "^A@B,1,1,ARI001^FT350,870^FD", w167, w203, w164, "^A@B,1,1,ARI001^FT380,870^FD", w168, w203, w164, "^A@B,1,1,ARI001^FT410,870^FD", w169, w203, w164, "^A@B,1,1,ARI001^FT440,870^FD", w170, w203, w164, "^A@B,1,1,ARI001^FT470,870^FD", w171, w203, w164, w164) -> (w194:string)
  n199 = Concatenate Strings("^A@B,1,1,ARI003.FNT^FT0,1060^FD", w138, w94, w86, w111, w94, w93, "^A@B,1,1,ARI003.FNT^FT40,1060^FD", w224, w94, w93, w99, w93, "^A@B,1,1,ARI003.FNT^FT80,1060^FD", w221, w94, w93, w95, w93, "^A@B,1,1,ARI003.FNT^FT120,1060^FD", w218, w94, w93, w92, w93, "^A@B,1,1,ARI003.FNT^FT200,1060^FD", w215, w94, w93, "^A@B,1,1,ARI003^FT235,990^FD(S/N)^FS", w93, w84, w93, w82, w93, w80, w93, w77, w93, w93) -> (w195:string)
  n200 = Concatenate Strings(w198, w125, w123, w41, w124, w123, w41, w122, w41, "^A@B,1,1,ARI002^FT660,800^FD", w197, w123, w41, w72, w175, w123, w41, "^A@B,1,1,ARI002^FT695,800^FD", w142, w123, w41, "^A@B,1,1,ARI005^FT695,680^FD", w141, w123, w41, w42, w41) -> (w193:string)
  n201 = Concatenate Strings(w119, "^XZ", w119) -> (w7:string)
  n202 = local read "DATA cmde"() -> (w6:T1)
  n203 = Unbundle By Name(w6) -> ("n°article FAS"=w4:string)
  n204 = Match Pattern(string=w4, regular expression="F120252") -> (offset past match=w2:i32)  [unwired: 1 in, 3 out]
  n205 = Greater Or Equal To 0?(x=w2) -> (x >= 0?=w1:bool)
  n206 = case shown="True" w1 {
    tunnel: ["" "^A@B,1,1,ARI005\n^FT500,760\n^FDSupplier Nb : MFG - 0001814\n^FS\n\n"] -> w5
    frame False {
    }
    frame True {
      # "Exception F120252 : imprimer numéro fournisseur"
    }
  }
  n207 = Concatenate Strings(w196, "^FT280,1060^GFA,03840,03840,00024,:Z64:\neJztlkEKgDAMBIMefLbfkb7KhwQjYi9Jc2ggYJDdS2EZ5tI0lCgrSzts0Z5jE9b9Ktd7+L3Dc5CHX/FDut/vHZ6DPPwTfqRmEubhF/NZz9/32y6nvi+/B/81X21+4CekbIb3Zf97pg/w/v6Ef9Jf6/3Cn7nHbknYBbU=:F74F" ("chaîne"), w195, w192, w194, w9, w193, w5, w7) -> (→"chaine  à écrire":string)
